vi "4Pi Focus Lock_v2.vi"() -> ()   [LabVIEW 2016]
uses:
  4Pi Focus Lock Controls/4Pi Focus Lock - Notifier Type.ctl
  4Pi Focus Lock Controls/4Pi Focus Lock - Actions.ctl
  <vilib>/vision/Image Controls.llb/IMAQ Image.ctl
  Hardware Configuration/Hardware Configuration Controls/Device Type.ctl
  Hardware Configuration/Hardware Configuration Controls/Device Function.ctl
  Device Library/Cameras/Camera Controls/Generic Camera ROI.ctl
  Device Library/Cameras/Camera Controls/Generic Camera Actions.ctl
  Device Library/Stages/Stages Controls/Stage Actions.ctl
  <vilib>/addons/control/pid/pid.llb/PID (DBL).vi
  <vilib>/addons/control/pid/NI_PID_pid.lvlib
  <vilib>/vision/NI_Vision_Development_Module.lvlib
panel:
  in  "Z Correction Active":bool=TRUE
  in  "Frame Accumulation":u32=1
  in  "Z Drift Threshold (µm)":dbl=2.0
  in  "Z Move Limit (µm)":dbl=2.0
  out "Z Move":bool
  in  "Update Scale Factor":dbl=2.0
  out "dz (µm)":dbl format="%.2f"
  out "dt (s)":dbl format="%.3f"
  out "Measured Z (µm)":dbl=1.0 format="%.3g"
  out "Target Z (µm)":dbl=1.0 format="%.3g"
  out "Stage Position (µm)":dbl=1.0 format="%.2g"
  in  "Quit":bool
  in  "Sample Z Step No.":u32=2
  in  "Sample Z Step Size (µm)":dbl=2.0
  in  "D (Derivative)":dbl
  in  "I (Integral)":dbl
  in  "P (Proportional)":dbl=2.0
  in  "Set Camera ROI":bool
  out "Z Target and Fit Value (µm)":T1(graph)
  in  "Start Lock":bool
  # "PID Control Values"
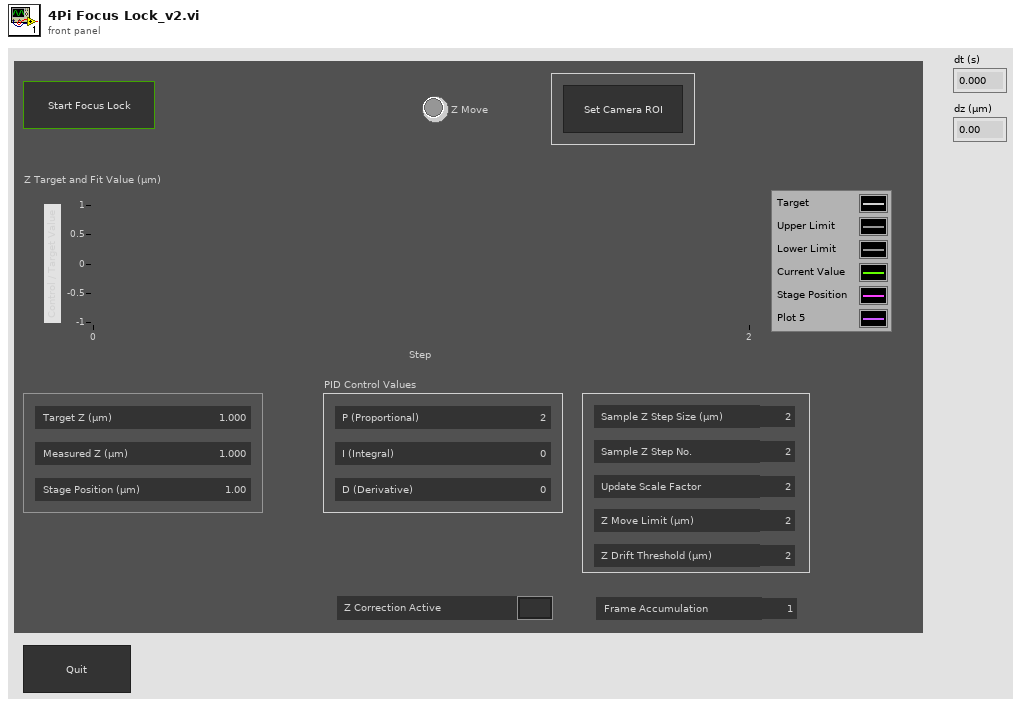
[diagram p1: front panel]
types:
  T1 = cluster{"Target 01":dbl, dbl, dbl, "Current 01":dbl, "Stage Position":dbl}
  T2 = typedef "4Pi Focus Lock - Actions.ctl" = enum16{"Idle", "Start Lock", "Restart Lock", "Get Target Position", "Get Ref Stack", "Cal Ref FFT", "Move To Init Z", "Start Primary Camera", "Get Current Position", "Get Current Position 1", "Get Actual Position", "Check Drift", "Move Z", "Update Plots", "Delay", "Abort", "Exit Loop", "Quit"}
  T3 = typedef "4Pi Focus Lock - Notifier Type.ctl" = cluster{"Actions":T2, "Z Drift Threshold":dbl, "Z Stage Move Limit (µm)":dbl, "Abort If Error":bool, "Z Correction Active":bool, "PID Values":dbl[], "Running?":bool, "Update Delay (ms)":i32, "Z Step Size (µm)":dbl, "Z Step No.":u32, "No. of Frames":u32, "Ref Stack (SGL)":T4[], "Cur Image (SGL)":T4, "CC Image (SGL) ":T4, "Sample Z (µm)":dbl[], "Initial Z Position (µm)":dbl, "Ref FFT Stack (CSG)":T4[], "Tmp Image FFT (CSG) ":T4[]}
  T4 = typedef "IMAQ Image.ctl" = refnum<image>
  T5 = typedef "Image Type" = u32
  T6 = typedef "Device Function.ctl" = enum16{"Primary", "Secondary", "Overview", "Wide Field Drift Correction", "642 nm Excitation", "560 nm Excitation", "940 nm Excitation", "546 nm Excitation", "488 nm Excitation", "405 nm Excitation", "Objective Drift Correction", "4Pi Focus Lock", "4Pi Objective Lock", "Objective XY", "Objective Z", "Sample XY", "Sample Coarse Z", "Sample Z", "4Pi Lower", "4Pi Upper", "Em Small", "Em Large", "Ex Small", "Ex Large", "Mojo", "Adj Cavity", "Line Scanning", "Alert"}
  T7 = typedef "Device Type.ctl" = enum16{"AOTF", "Camera", "Deformable Mirror", "Laser", "Flip Mirror", "Shutter", "Stage", "Waveform", "FPGA", "Email"}
  T8 = typedef "Stage Actions.ctl" = enum16{"Get Position", "MVR", "MOVE", "HALT", "ONTARGET", "ERROR", "REFERENCE", "INIT", "VELOCITY", "STATUS", "EXIT", "HOME", "ZEROPOS", "NANOPOS", "ANALOG", "QUIT"}
  T9 = typedef "Generic Camera Actions.ctl" = enum16{"Status", "Live Preview", "Capture", "Abort", "Set Exposure Time (s)", "Get Exposure Time (s)", "Record Settings", "Set ROI", "Get ROI", "Defect Correction On/Off", "Cooler On/Off", "Fan On/Off", "Quit"}
  T10 = typedef "Generic Camera ROI.ctl" = cluster{"H_Offset":u16, "V_Offset":u16, "H_Width":u16, "V_Width":u16}
  T11 = typedef "Stage Status.ctl" = enum16{"Error", "Abort", "Busy", "On Target"}
  T12 = cluster{"PID Values[0]":dbl, "PID Values[1]":dbl, "PID Values[2]":dbl}
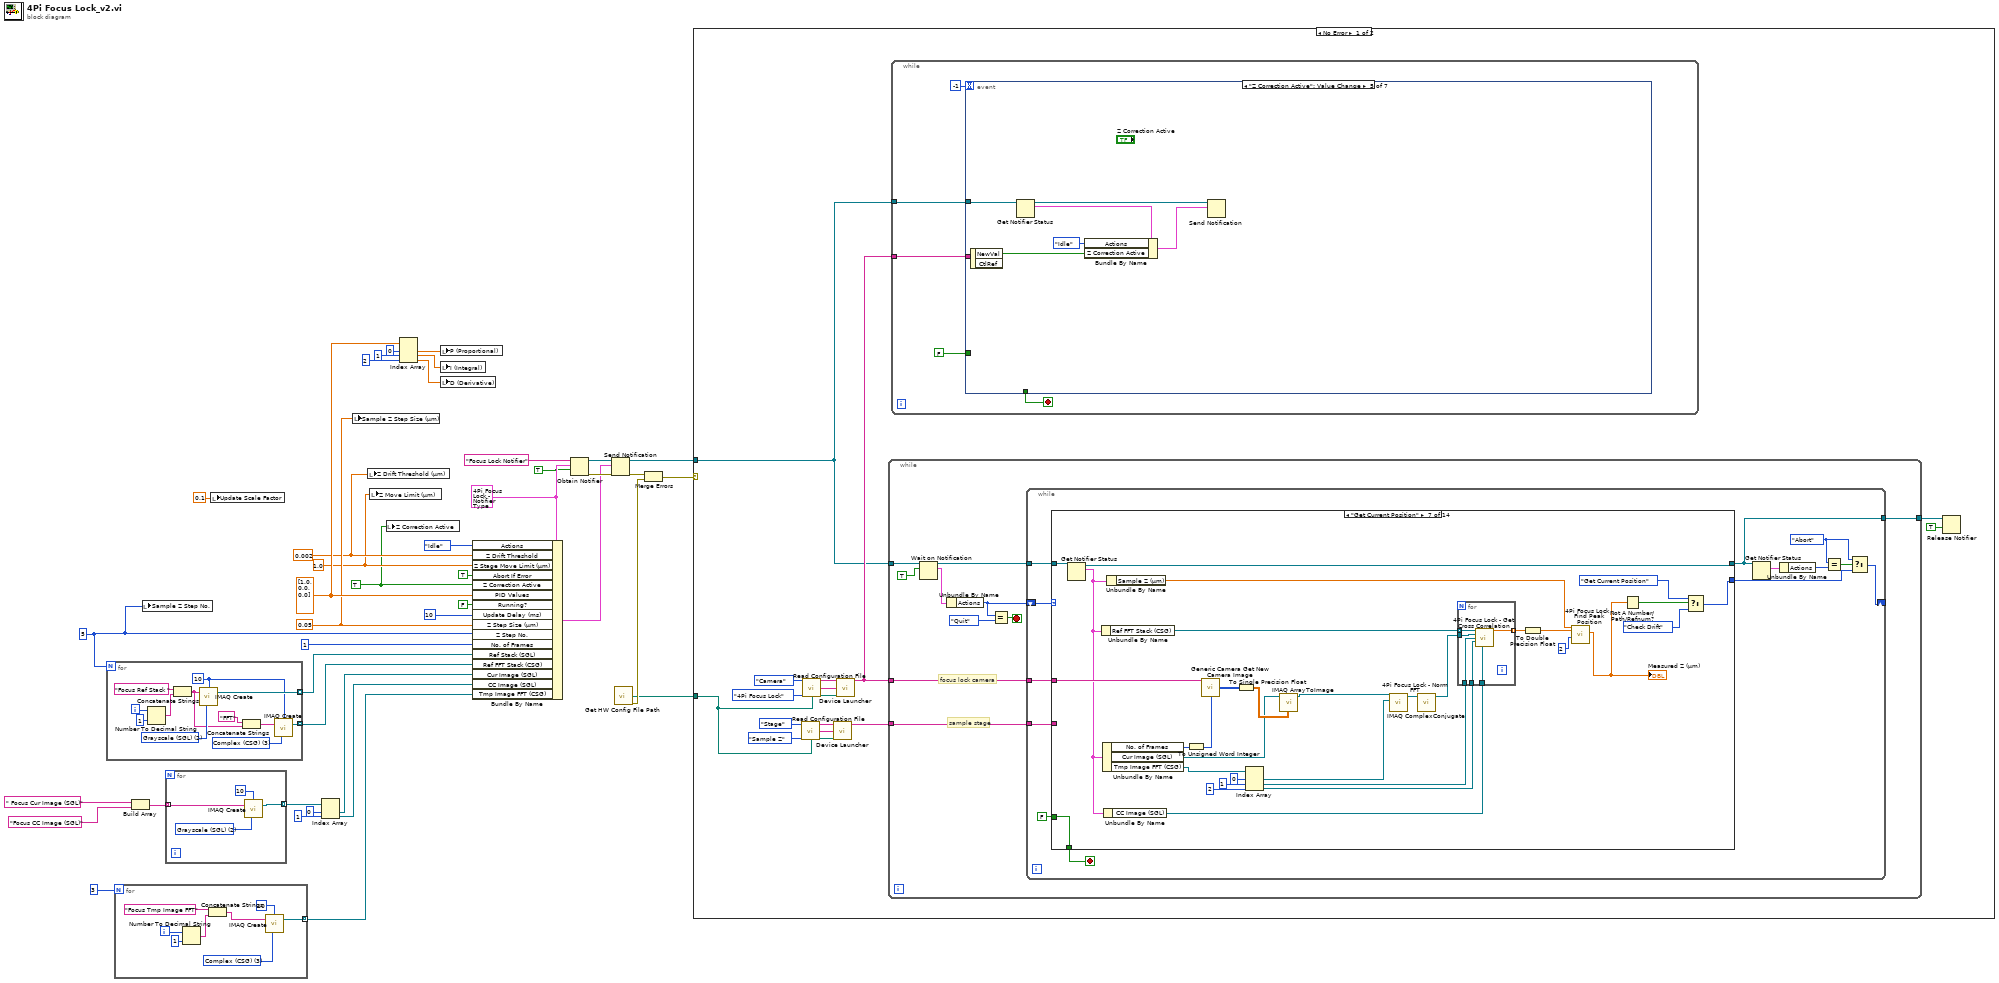
[diagram p0: block diagram]
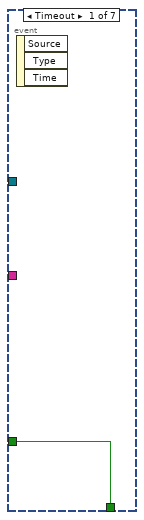
[diagram p2: hidden frame]
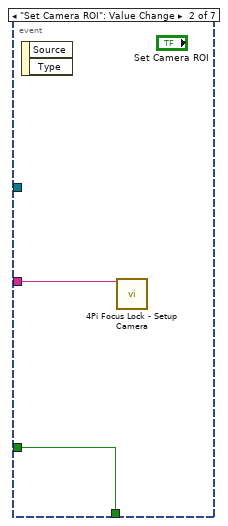
[diagram p3: hidden frame]
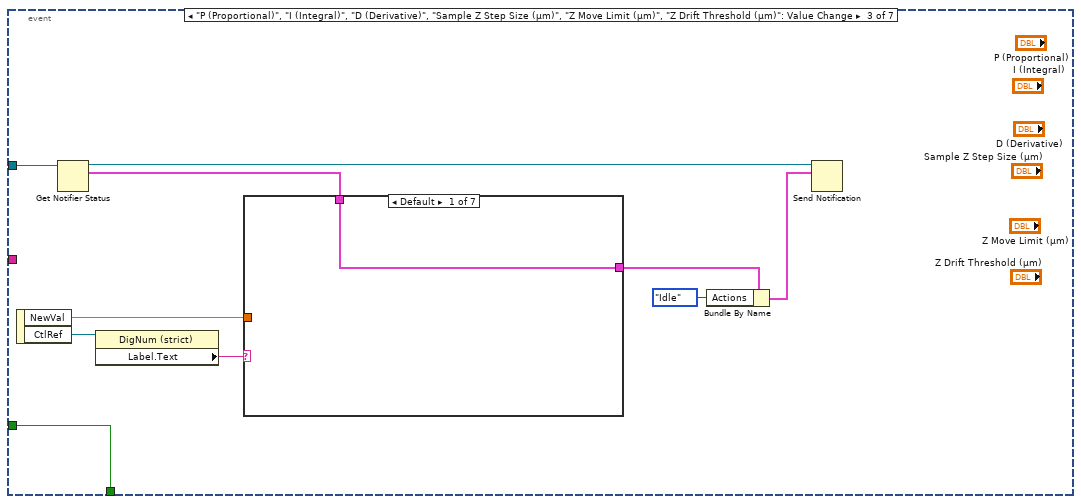
[diagram p4: hidden frame]
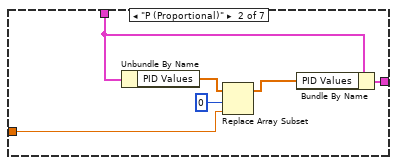
[diagram p5: hidden frame]
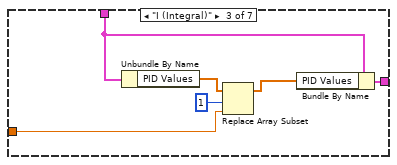
[diagram p6: hidden frame]
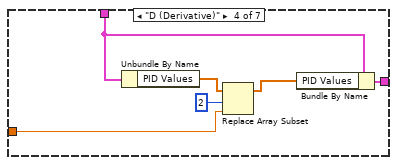
[diagram p7: hidden frame]
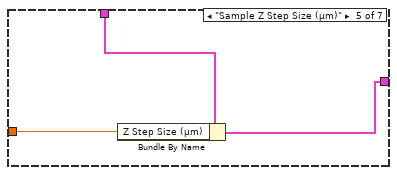
[diagram p8: hidden frame]
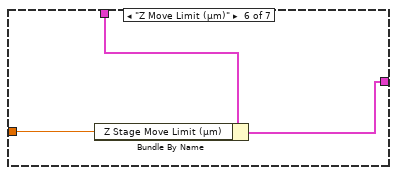
[diagram p9: hidden frame]
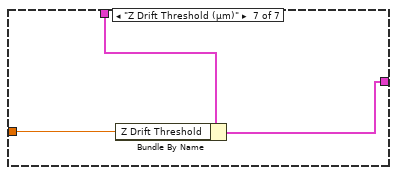
[diagram p10: hidden frame]
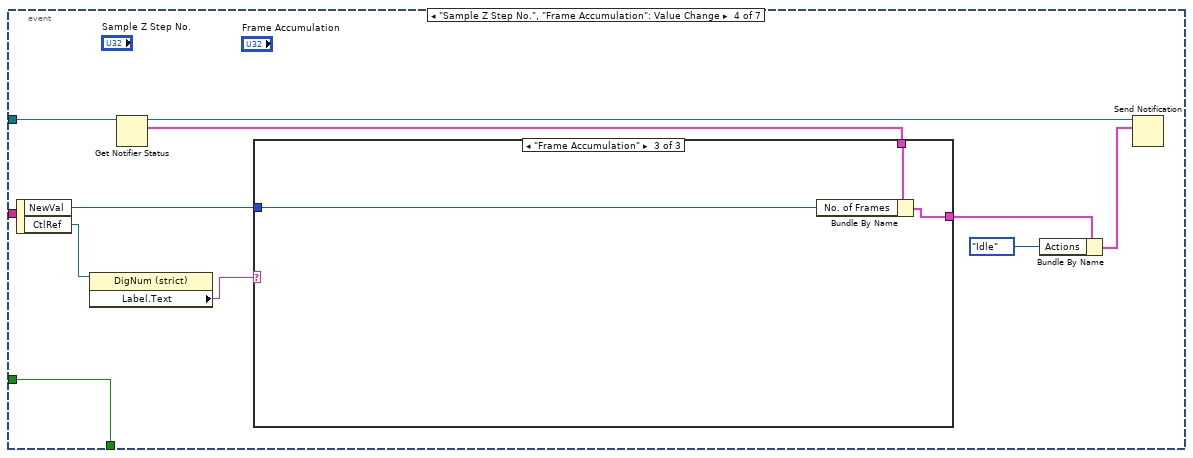
[diagram p11: hidden frame]
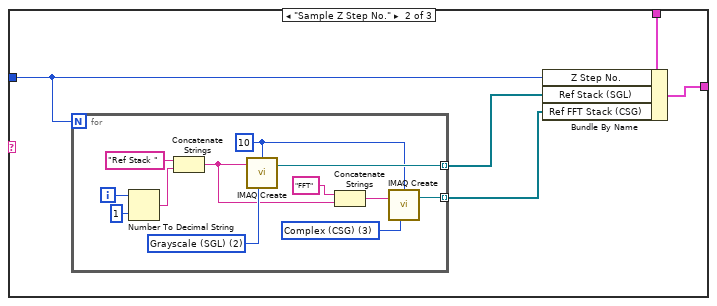
[diagram p13: hidden frame]
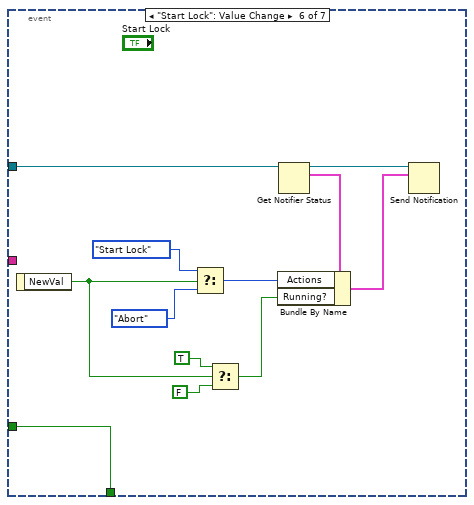
[diagram p14: hidden frame]
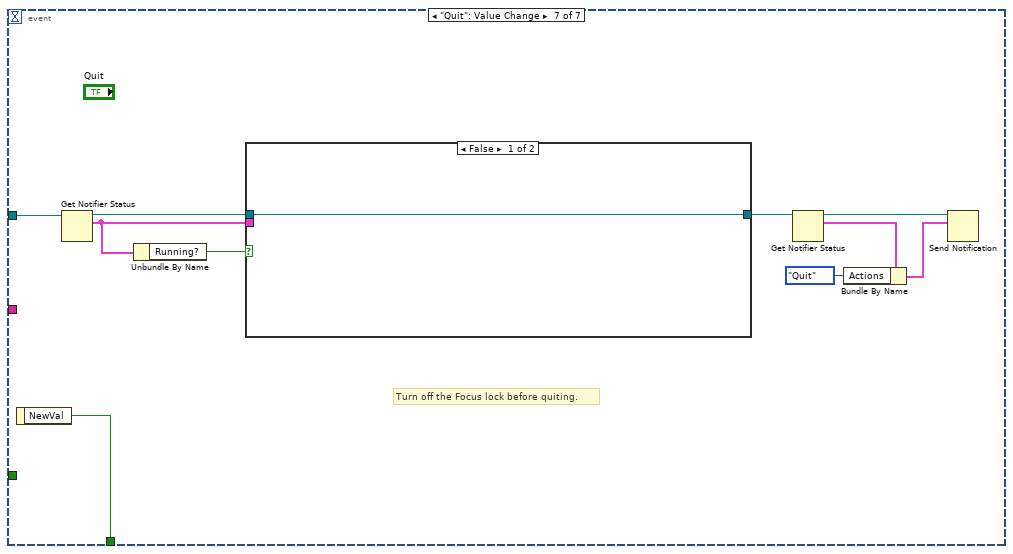
[diagram p15: hidden frame]
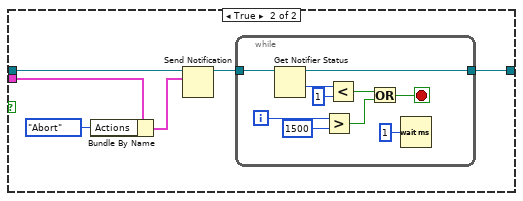
[diagram p16: hidden frame]
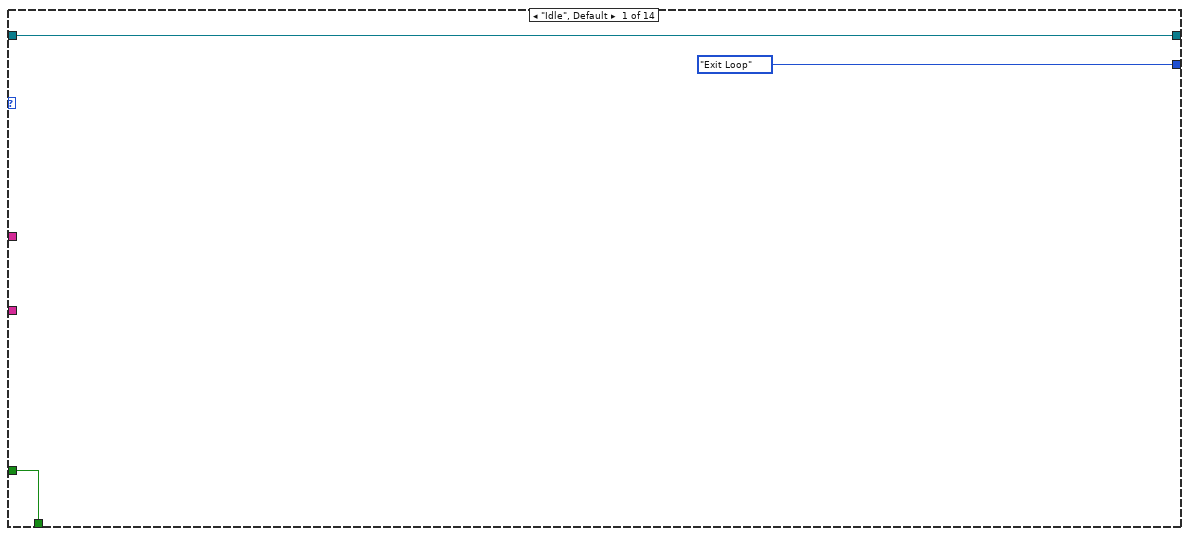
[diagram p17: hidden frame]
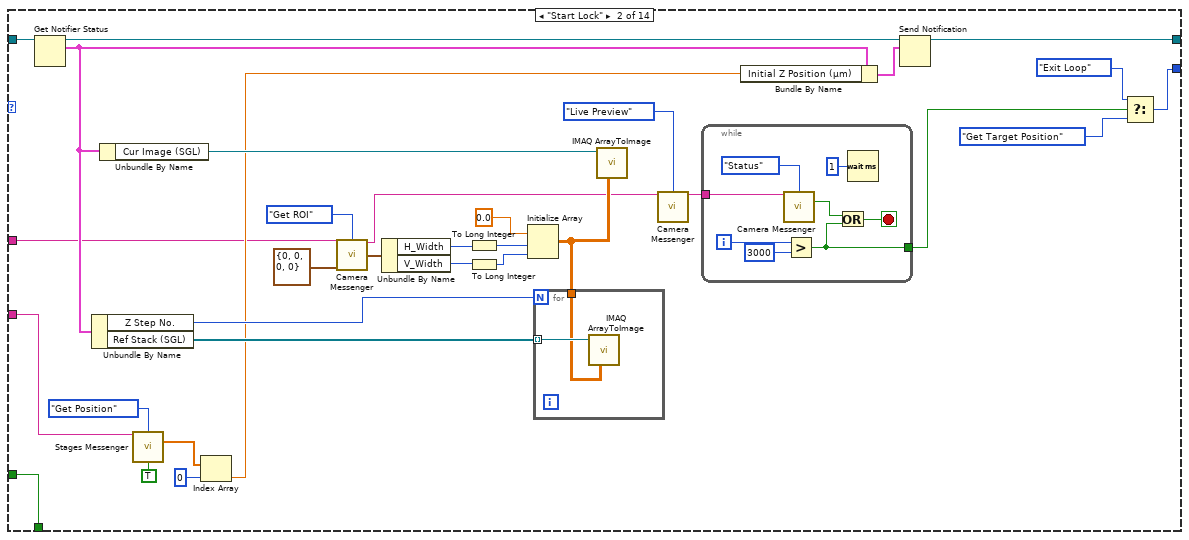
[diagram p18: hidden frame]
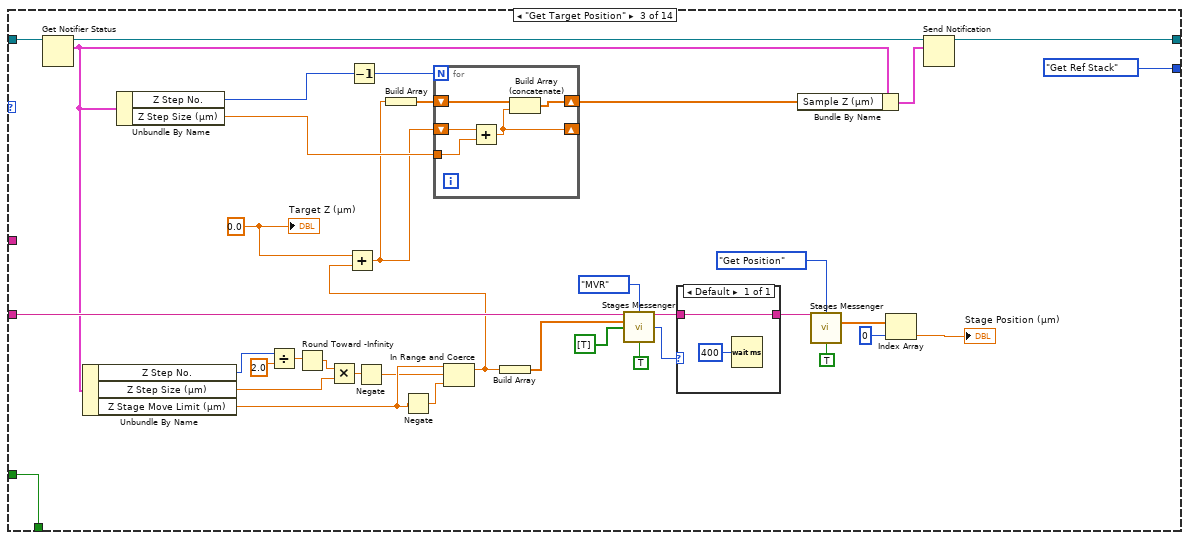
[diagram p19: hidden frame]
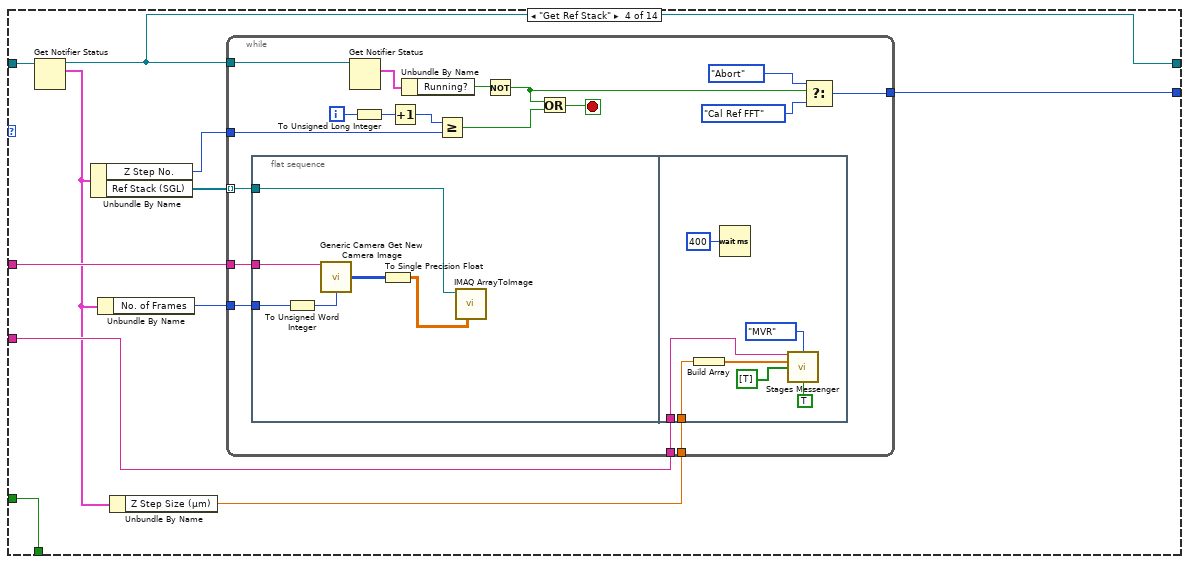
[diagram p20: hidden frame]
diagram:
  w20 = u32 5 ("Z Step No.")
  w27 = 0.05 ("Z Step Size (µm)")
  w31 = dbl[] [1.0, 0.0, 0.0] ("PID Values")
  w1 = TRUE ("Z Correction Active")
  w7 = 1.0 ("Z Stage Move Limit (µm)")
  w8 = 0.002 ("Z Drift Threshold")
  w10 = T3 {"Actions"=enum."Idle", "Z Drift Threshold"=0.05, "Z Stage Move Limit (µm)"=1.0, "Abort If Error"=FALSE, "Z Correction Active"=FALSE, "PID Values"=[], "Running?"=FALSE, "Update Delay (ms)"=0, "Z Step Size (µm)"=2.0, "Z Step No."=2, "No. of Frames"=0, "Ref Stack (SGL)"=[], "Cur Image (SGL)"=refnum, "CC Image (SGL) "=refnum, "Sample Z (µm)"=[], "Initial Z Position (µm)"=0.0, "Ref FFT Stack (CSG)"=[], "Tmp Image FFT (CSG) "=[]} ("4Pi Focus Lock")
  n1 = for {
    N: w20 -> [_]
    tunnel: [w53] -> w19 mode=indexing
    tunnel: [w42] -> w4 mode=indexing
    i -> [w52]
    w47 = T5 3 items=["Grayscale (U8)", "Grayscale (I16)", "Grayscale (SGL)", "Complex (CSG)", "RGB (U32)", "HSL (U32)", "RGB (U64)", "Grayscale (U16)"] ("Image Type")
    w48 = T5 2 items=["Grayscale (U8)", "Grayscale (I16)", "Grayscale (SGL)", "Complex (CSG)", "RGB (U32)", "HSL (U32)", "RGB (U64)", "Grayscale (U16)"] ("Image Type")
    w44 = 10 ("Border Size")
    n2 = Number To Decimal String(number=w52, width (-)=i16 1) -> (decimal integer string=w50:string)
    n3 = Concatenate Strings("Focus Ref Stack " ("string"), w50) -> (w43:string)
    n4 = call "IMAQ Create"("Border Size"=w44, "Image Name"=w43, "Image Type"=w48) -> ("New Image"=w53:T4)  [unwired: 2 in, 1 out]
    n5 = Concatenate Strings("FFT" ("string"), w43) -> (w46:string)
    n6 = call "IMAQ Create"("Border Size"=w44, "Image Name"=w46, "Image Type"=w47) -> ("New Image"=w42:T4)  [unwired: 2 in, 1 out]
  }
  n7 = for {
    N: 3 -> [_]
    tunnel: [w59] -> w2 mode=indexing
    i -> [w55]
    w60 = T5 3 items=["Grayscale (U8)", "Grayscale (I16)", "Grayscale (SGL)", "Complex (CSG)", "RGB (U32)", "HSL (U32)", "RGB (U64)", "Grayscale (U16)"] ("Image Type")
    n8 = Number To Decimal String(number=w55, width (-)=i16 1) -> (decimal integer string=w58:string)
    n9 = Concatenate Strings("Focus Tmp Image FFT" ("Image Name"), w58) -> (w54:string)
    n10 = call "IMAQ Create"("Border Size"=10, "Image Name"=w54, "Image Type"=w60) -> ("New Image"=w59:T4)  [unwired: 2 in, 1 out]
  }
  n11 = Build Array(" Focus Cur Image (SGL)" ("Image Name"), "Focus CC Image (SGL)" ("Image Name")) -> (w14:string[])
  n12 = local write "Sample Z Step No."(w20) -> ()
  n13 = for {
    tunnel: w14 -> [w63] mode=indexing
    tunnel: [w62] -> w13 mode=indexing
    w64 = T5 2 items=["Grayscale (U8)", "Grayscale (I16)", "Grayscale (SGL)", "Complex (CSG)", "RGB (U32)", "HSL (U32)", "RGB (U64)", "Grayscale (U16)"] ("Image Type")
    n14 = call "IMAQ Create"("Border Size"=10, "Image Name"=w63, "Image Type"=w64) -> ("New Image"=w62:T4)  [unwired: 2 in, 1 out]
  }
  n15 = local write "Update Scale Factor"(0.1 ("Update Scale Factor")) -> ()
  n16 = Index Array(array=w13, index #1=0 ("index"), index #2=1 ("index")) -> (element #1=w12:T4, element #2=w11:T4)
  n17 = local write "Sample Z Step Size (µm)"(w27) -> ()
  n18 = local write "Z Drift Threshold (µm)"(w8) -> ()
  n19 = local write "Z Move Limit (µm)"(w7) -> ()
  n20 = local write "Z Correction Active"(w1) -> ()
  n21 = Index Array(array=w31, index #1=0 ("index"), index #2=1 ("index"), index #3=2 ("index")) -> (element #1=w30:dbl, element #2=w29:dbl, element #3=w28:dbl)
  n22 = local write "P (Proportional)"(w30) -> ()
  n23 = local write "I (Integral)"(w29) -> ()
  n24 = local write "D (Derivative)"(w28) -> ()
  n25 = Bundle By Name(cluster=w10, "Actions"=4Pi_Focus_Lock_-_Actions."Idle", "Z Drift Threshold"=w8, "Z Stage Move Limit (µm)"=w7, "Abort If Error"=TRUE, "Z Correction Active"=w1, "PID Values"=w31, "Running?"=FALSE, "Update Delay (ms)"=10, "Z Step Size (µm)"=w27, "Z Step No."=w20, "No. of Frames"=u32 1, "Ref Stack (SGL)"=w19, "Ref FFT Stack (CSG)"=w4, "Cur Image (SGL)"=w12, "CC Image (SGL)"=w11, "Tmp Image FFT (CSG)"=w2) -> (w5:T3)
  n26 = Obtain Notifier(name (unnamed)="Focus Lock Notifier", notification data type=w10, create if not found? (T)=TRUE) -> (notifier out=w36:refnum<notifier>, error out=w35:errorcluster)  [unwired: 1 in, 1 out]
  n27 = Send Notification(notification=w5, notifier=w36, error in (no error)=w35) -> (notifier out=w22:refnum<notifier>, error out=w26:errorcluster)
  n28 = call "Get HW Config File Path.vi"() -> ("File Path"=w24:path, "Error"=w25:errorcluster)  [unwired: 14 in]
  n29 = Merge Errors(w26, w25) -> (w23:errorcluster)
  n30 = case shown="No Error" w23 {
    tunnel: w24 -> [w66 _]
    tunnel: w22 -> [w69 _]
    frame No Error {
      n31 = call "Read Configuration File.vi"("Device Type"=Device_Type."Stage", "Device Function"=Device_Function."Sample Z", "Config File Path"=w66) -> ("Unique Notifier Name"=w76:string, "Device Ports/IDs/Channels"=w74:string[], "Device Engine Path"=w73:path)  [unwired: 9 in, 1 out]
      n32 = call "Read Configuration File.vi"("Device Type"=Device_Type."Camera", "Device Function"=Device_Function."4Pi Focus Lock", "Config File Path"=w66) -> ("Unique Notifier Name"=w81:string, "Device Ports/IDs/Channels"=w80:string[], "Device Engine Path"=w79:path)  [unwired: 9 in, 1 out]
      n33 = call "Device Launcher.vi"("Notifier Name"=w76, "Device Ports/IDs/Channels"=w74, "Device Engine Path"=w73) -> ("Notifier Name"=w71:string)  [unwired: 11 in, 1 out]
      n34 = call "Device Launcher.vi"("Notifier Name"=w81, "Device Ports/IDs/Channels"=w80, "Device Engine Path"=w79) -> ("Notifier Name"=w70:string)  [unwired: 11 in, 1 out]
      n35 = while {
        tunnel: w69 -> [w213]
        tunnel: w70 -> [w207]
        tunnel: w71 -> [w206]
        tunnel: [w204] -> w67
        stop <- w209 stop-if-true
        # "sample stage"
        # "focus lock camera"
        n36 = Wait on Notification(notifier=w213, ignore previous (F)=TRUE) -> (notifier out=w205:refnum<notifier>, notification=w211:T3)  [unwired: 2 in, 2 out]
        n37 = Unbundle By Name(w211) -> ("Actions"=w208:T2)
        n38 = Equal?(x=w208, y=4Pi_Focus_Lock_-_Actions."Quit") -> (x = y?=w209:bool)
        n39 = while {
          tunnel: w207 -> [w225]
          tunnel: w206 -> [w224]
          tunnel: w205 -> [w223]
          shift-right: [w217] -> _
          shift-left: w208 -> [w226]
          tunnel: [w214] -> w204
          stop <- w216 stop-if-true
          w219 = 4Pi_Focus_Lock_-_Actions."Abort" ("y")
          n40 = case shown="\"Get Current Position\"" w226 {
            tunnel: w225 -> [_ w236 _ w325 _ _ w404 w432 _ _ _ w527 _ _]
            tunnel: w224 -> [_ w244 w303 w318 _ w370 _ _ _ w491 w510 _ _ _]
            tunnel: w223 -> [w227 w254 w304 w326 w363 w375 w421 w447 w476 w496 w520 w528 w535 w538]
            tunnel: [4Pi_Focus_Lock_-_Actions."Exit Loop" ("y") w230 4Pi_Focus_Lock_-_Actions."Get Ref Stack" ("y") w319 4Pi_Focus_Lock_-_Actions."Move To Init Z" ("y") 4Pi_Focus_Lock_-_Actions."Get Current Position" ("y") w407 4Pi_Focus_Lock_-_Actions."Check Drift" ("y") w459 w481 4Pi_Focus_Lock_-_Actions."Get Current Position" ("y") 4Pi_Focus_Lock_-_Actions."Exit Loop" ("y") 4Pi_Focus_Lock_-_Actions."Exit Loop" ("y") 4Pi_Focus_Lock_-_Actions."Quit" ("y")] -> w218
            tunnel: [w227 w239 w291 w321 w360 w373 w417 w442 w469 w489 w508 w524 w535 w538] -> w214
            tunnel: [w228 w238 w290 w320 w358 w371 w416 w441 w468 w488 w507 w523 TRUE TRUE] -> w216
            tunnel: FALSE -> [w228 w238 w290 w320 w358 w371 w416 w441 w468 w488 w507 w523 _ _]
            frame "Idle", Default {
            }
            frame "Start Lock" {
              n41 = Get Notifier Status(notifier=w254) -> (notifier out=w240:refnum<notifier>, current notification=w243:T3)  [unwired: 1 in, 3 out]
              n42 = Unbundle By Name(w243) -> ("Z Step No."=w251:u32, "Ref Stack (SGL)"=w250:T4[])
              n43 = Unbundle By Name(w243) -> ("Cur Image (SGL)"=w248:T4)
              n44 = call "Stages Messenger.vi"("Stage Notifier Name"=w244, "Actions"=Stage_Actions."Get Position", "Exit While Busy?"=TRUE) -> ("Positions"=w245:dbl[])  [unwired: 9 in, 3 out]
              n45 = Index Array(array=w245, index=0) -> (element=w242:dbl)
              n46 = call "Camera Messenger.vi"("Notifier Name"=w236, "General Camera Actions"=Generic_Camera_Actions."Get ROI", "Camera ROI"=T10 {"H_Offset"=0, "V_Offset"=0, "H_Width"=0, "V_Width"=0} ("General Camera ROI")) -> ("Notifier Name Dup"=w235:string, "Camera ROI"=w259:T10)  [unwired: 7 in, 4 out]
              n47 = Unbundle By Name(w259) -> ("H_Width"=w258:u16, "V_Width"=w256:u16)
              n48 = To Long Integer(number=w258) -> (32bit integer=w257:i32)
              n49 = To Long Integer(number=w256) -> (32bit integer=w255:i32)
              n50 = Initialize Array(sgl 0.0 ("element"), w257, w255) -> (w249:sgl[][])
              n51 = for {
                N: w251 -> [_]
                tunnel: w249 -> [w270]
                tunnel: w250 -> [w271] mode=indexing
                n52 = call "IMAQ ArrayToImage"("Image Pixels (Float)"=w270, "Image"=w271) -> ()  [unwired: 8 in, 2 out]
              }
              n53 = call "IMAQ ArrayToImage"("Image Pixels (Float)"=w249, "Image"=w248) -> ()  [unwired: 8 in, 2 out]
              n54 = call "Camera Messenger.vi"("Notifier Name"=w235, "General Camera Actions"=Generic_Camera_Actions."Live Preview") -> ("Notifier Name Dup"=w234:string)  [unwired: 8 in, 5 out]
              n55 = while {
                tunnel: w234 -> [w268]
                tunnel: [w263] -> w233
                i -> [w267]
                stop <- w264 stop-if-true
                n56 = call "Camera Messenger.vi"("Notifier Name"=w268, "General Camera Actions"=Generic_Camera_Actions."Status") -> ("Running?"=w265:bool)  [unwired: 8 in, 5 out]
                n57 = Greater?(x=w267, y=3000) -> (0:w263:bool)
                n58 = Or(x=w265, y=w263) -> (x .or. y?=w264:bool)
                n59 = Wait (ms)(milliseconds to wait=u32 1) -> ()  [unwired: 1 out]
              }
              n60 = Bundle By Name(cluster=w243, "Initial Z Position (µm)"=w242) -> (w241:T3)
              n61 = Send Notification(notification=w241, notifier=w240) -> (notifier out=w239:refnum<notifier>)  [unwired: 1 in, 1 out]
              n62 = Select(t=4Pi_Focus_Lock_-_Actions."Exit Loop" ("y"), s=w233, f=4Pi_Focus_Lock_-_Actions."Get Target Position") -> (s? t:f=w230:T2)
            }
            frame "Get Target Position" {
              w297 = 0.0 ("Target Z (µm)")
              n63 = Get Notifier Status(notifier=w304) -> (notifier out=w295:refnum<notifier>, current notification=w300:T3)  [unwired: 1 in, 3 out]
              n64 = Unbundle By Name(w300) -> ("Z Step No."=w289:u32, "Z Step Size (µm)"=w288:dbl, "Z Stage Move Limit (µm)"=w286:dbl)
              n65 = Unbundle By Name(w300) -> ("Z Step No."=w281:u32, "Z Step Size (µm)"=w298:dbl)
              n66 = Divide(x=w289, y=2.0) -> (x/y=w279:dbl)
              n67 = Round Toward -Infinity(1:w279) -> (0:w278:dbl)
              n68 = Multiply(x=w278, y=w288) -> (x*y=w283:dbl)
              n69 = Decrement(x=w281) -> (x-1=w280:u32)
              n70 = Negate(x=w283) -> (-x=w282:dbl)
              n71 = Negate(x=w286) -> (-x=w287:dbl)
              n72 = In Range and Coerce(upper limit=w286, x=w282, lower limit=w287) -> (coerced(x)=w284:dbl)  [unwired: 1 out]
              n73 = Add(x=w297, y=w284) -> (x+y=w285:dbl)
              n74 = Build Array(w285) -> (w299:dbl[])
              n75 = for {
                N: w280 -> [_]
                tunnel: w298 -> [w313]
                shift-right: [w314] -> w296
                shift-left: w299 -> [w315]
                shift-right: [w311] -> _
                shift-left: w285 -> [w312]
                n76 = Add(x=w312, y=w313) -> (x+y=w311:dbl)
                n77 = Build Array (concatenate)(w315, w311) -> (w314:dbl[])
              }
              n78 = Build Array(w284) -> (w301:dbl[])
              n79 = call "Stages Messenger.vi"("Stage Notifier Name"=w303, "Actions"=Stage_Actions."MVR", "Setpoint"=w301, "Axis"=bool[] [TRUE], "Exit While Busy?"=TRUE) -> ("Stage Notifier Name (Dup)"=w276:string, "Status"=w277:T11)  [unwired: 7 in, 2 out]
              n80 = case shown="Default" w277 {
                tunnel: [w309] -> w275
                tunnel: w276 -> [w309]
                frame Default {
                  n81 = Wait (ms)(milliseconds to wait=u32 400) -> ()  [unwired: 1 out]
                }
              }
              n82 = Bundle By Name(cluster=w300, "Sample Z (µm)"=w296) -> (w294:T3)
              n83 = call "Stages Messenger.vi"("Stage Notifier Name"=w275, "Actions"=Stage_Actions."Get Position", "Exit While Busy?"=TRUE) -> ("Positions"=w273:dbl[])  [unwired: 9 in, 3 out]
              n84 = Index Array(array=w273, index=0) -> (element=→"Stage Position (µm)":dbl)
              n85 = Send Notification(notification=w294, notifier=w295) -> (notifier out=w291:refnum<notifier>)  [unwired: 1 in, 1 out]
              "Target Z (µm)" <- w297
            }
            frame "Get Ref Stack" {
              n86 = Get Notifier Status(notifier=w326) -> (notifier out=w321:refnum<notifier>, current notification=w317:T3)  [unwired: 1 in, 3 out]
              n87 = Unbundle By Name(w317) -> ("Z Step No."=w324:u32, "Ref Stack (SGL)"=w323:T4[])
              n88 = Unbundle By Name(w317) -> ("No. of Frames"=w316:u32)
              n89 = Unbundle By Name(w317) -> ("Z Step Size (µm)"=w322:dbl)
              n90 = while {
                tunnel: w325 -> [w344]
                tunnel: w324 -> [w341]
                tunnel: w321 -> [w343]
                tunnel: [w331] -> w319
                tunnel: w323 -> [w330] mode=indexing
                tunnel: w322 -> [w329]
                tunnel: w318 -> [w328]
                tunnel: w316 -> [w327]
                i -> [w340]
                stop <- w336 stop-if-true
                n91 = flat-sequence {
                  tunnel: w344 -> [w348]
                  tunnel: w330 -> [w347]
                  tunnel: w327 -> [w346]
                  tunnel: w329 -> [w352]
                  tunnel: w328 -> [w351]
                  frame #0 {
                    n92 = To Unsigned Word Integer(number=w346) -> (unsigned 16bit integer=w345:u16)
                    n93 = call "Generic Camera Get New Camera Image.vi"("Camera Notifier Name"=w348, "Frames"=w345) -> ("Image - U16"=w350:u16[][])  [unwired: 11 in, 2 out]
                    n94 = To Single Precision Float(number=w350) -> (single precision float=w349:sgl[][])
                    n95 = call "IMAQ ArrayToImage"("Image Pixels (Float)"=w349, "Image"=w347) -> ()  [unwired: 8 in, 2 out]
                  }
                  frame #1 {
                    n96 = Build Array(w352) -> (w356:dbl[])
                    n97 = Wait (ms)(milliseconds to wait=u32 400) -> ()  [unwired: 1 out]
                    n98 = call "Stages Messenger.vi"("Stage Notifier Name"=w351, "Actions"=Stage_Actions."MVR", "Setpoint"=w356, "Axis"=bool[] [TRUE], "Exit While Busy?"=TRUE) -> ()  [unwired: 7 in, 4 out]
                  }
                }
                n99 = Get Notifier Status(notifier=w343) -> (current notification=w335:T3)  [unwired: 1 in, 4 out]
                n100 = To Unsigned Long Integer(number=w340) -> (unsigned 32bit integer=w339:u32)
                n101 = Increment(x=w339) -> (x+1=w342:u32)
                n102 = Unbundle By Name(w335) -> ("Running?"=w338:bool)
                n103 = Greater Or Equal?(x=w342, y=w341) -> (x >= y?=w337:bool)
                n104 = Not(x=w338) -> (.not. x?=w334:bool)
                n105 = Or(x=w334, y=w337) -> (x .or. y?=w336:bool)
                n106 = Select(t=4Pi_Focus_Lock_-_Actions."Abort", s=w334, f=4Pi_Focus_Lock_-_Actions."Cal Ref FFT" ("y")) -> (s? t:f=w331:T2)
              }
            }
            frame "Cal Ref FFT" {
              n107 = Get Notifier Status(notifier=w363) -> (notifier out=w360:refnum<notifier>, current notification=w364:T3)  [unwired: 1 in, 3 out]
              n108 = Unbundle By Name(w364) -> ("Ref Stack (SGL)"=w361:T4[], "Ref FFT Stack (CSG)"=w362:T4[])
              n109 = for {
                tunnel: w362 -> [w365] mode=indexing
                tunnel: w361 -> [w366] mode=indexing
                n110 = call "4Pi Focus Lock - Norm FFT.vi"("FFT Image Dst"=w365, "Image In"=w366) -> ()  [unwired: 8 in, 2 out]
              }
            }
            frame "Move To Init Z" {
              n111 = Get Notifier Status(notifier=w375) -> (notifier out=w373:refnum<notifier>, current notification=w374:T3)  [unwired: 1 in, 3 out]
              n112 = Unbundle By Name(w374) -> ("Initial Z Position (µm)"=w368:dbl)
              n113 = flat-sequence {
                tunnel: w370 -> [w383]
                tunnel: [w382] -> w369
                tunnel: w368 -> [w378]
                tunnel: [w376] -> w367
                tunnel: w369 -> [w387]
                tunnel: w367 -> [w386]
                frame #0 {
                  n114 = call "Stages Messenger.vi"("Stage Notifier Name"=w383, "Actions"=Stage_Actions."Get Position") -> ("Stage Notifier Name (Dup)"=w382:string, "Positions"=w380:dbl[])  [unwired: 10 in, 2 out]
                  n115 = Index Array(array=w380, index=0) -> (element=w379:dbl)
                  n116 = Subtract(x=w378, y=w379) -> (x-y=w377:dbl)
                  n117 = Build Array(w377) -> (w376:dbl[])
                }
                frame #1 {
                  n118 = Wait (ms)(milliseconds to wait=u32 400) -> ()  [unwired: 1 out]
                  n119 = call "Stages Messenger.vi"("Stage Notifier Name"=w387, "Actions"=Stage_Actions."MVR", "Setpoint"=w386, "Axis"=bool[] [TRUE], "Exit While Busy?"=TRUE) -> ()  [unwired: 7 in, 4 out]
                }
              }
            }
            frame "Get Current Position" {
              n120 = Get Notifier Status(notifier=w421) -> (notifier out=w417:refnum<notifier>, current notification=w401:T3)  [unwired: 1 in, 3 out]
              n121 = Unbundle By Name(w401) -> ("Ref FFT Stack (CSG)"=w415:T4[])
              n122 = Unbundle By Name(w401) -> ("No. of Frames"=w392:u32, "Cur Image (SGL)"=w403:T4, "Tmp Image FFT (CSG)"=w397:T4[])
              n123 = Unbundle By Name(w401) -> ("CC Image (SGL)"=w393:T4)
              n124 = Unbundle By Name(w401) -> ("Sample Z (µm)"=w419:dbl[])
              n125 = To Unsigned Word Integer(number=w392) -> (unsigned 16bit integer=w391:u16)
              n126 = call "Generic Camera Get New Camera Image.vi"("Camera Notifier Name"=w404, "Frames"=w391) -> ("Image - U16"=w406:u16[][])  [unwired: 11 in, 2 out]
              n127 = To Single Precision Float(number=w406) -> (single precision float=w405:sgl[][])
              n128 = Index Array(array=w397, index #1=0 ("index"), index #2=1 ("index"), index #3=2 ("index")) -> (element #1=w396:T4, element #2=w395:T4, element #3=w394:T4)
              n129 = call "IMAQ ArrayToImage"("Image Pixels (Float)"=w405, "Image"=w403) -> ("Image Out"=w402:T4)  [unwired: 8 in, 1 out]
              n130 = call "4Pi Focus Lock - Norm FFT.vi"("FFT Image Dst"=w396, "Image In"=w402) -> ("FFT Image Out"=w413:T4)  [unwired: 8 in, 1 out]
              n131 = call "IMAQ ComplexConjugate"("Image Src"=w413) -> ("Image Dst Out"=w412:T4)  [unwired: 3 in, 1 out]
              n132 = for {
                tunnel: w393 -> [w427]
                tunnel: [w426] -> w420 mode=indexing
                tunnel: w412 -> [w425]
                tunnel: w415 -> [w424] mode=indexing
                tunnel: w394 -> [w423]
                tunnel: w395 -> [w422]
                n133 = call "4Pi Focus Lock - Get Cross Correlation.vi"("Ref FFT image"=w424, "Cur FFT Image"=w425, "FFT CC image"=w422, "iFFT image"=w423, "CC image"=w427) -> ("Max CC"=w426:sgl)  [unwired: 9 in, 1 out]
              }
              n134 = To Double Precision Float(number=w420) -> (double precision float=w414:dbl[])
              n135 = call "4Pi Focus Lock - Find Peak Position.vi"("Fit Size"=2, "y"=w414, "x"=w419) -> ("Coerced Peak Position"=w411:dbl)  [unwired: 7 in, 1 out]
              "Measured Z (µm)" <- w411
              n136 = Not A Number/Path/Refnum?(number/path/refnum=w411) -> (NaN/Path/Refnum?=w410:bool)
              n137 = Select(t=4Pi_Focus_Lock_-_Actions."Get Current Position", s=w410, f=4Pi_Focus_Lock_-_Actions."Check Drift" ("y")) -> (s? t:f=w407:T2)
            }
            frame "Get Current Position 1" {
              n138 = Get Notifier Status(notifier=w447) -> (notifier out=w442:refnum<notifier>, current notification=w446:T3)  [unwired: 1 in, 3 out]
              n139 = Unbundle By Name(w446) -> ("No. of Frames"=w429:u32, "Cur Image (SGL)"=w431:T4, "CC Image (SGL)"=w437:T4)
              n140 = Unbundle By Name(w446) -> ("Sample Z (µm)"=w445:dbl[])
              n141 = Unbundle By Name(w446) -> ("Ref Stack (SGL)"=w440:T4[])
              n142 = To Unsigned Word Integer(number=w429) -> (unsigned 16bit integer=w428:u16)
              n143 = call "Generic Camera Get New Camera Image.vi"("Camera Notifier Name"=w432, "Frames"=w428) -> ("Image - U16"=w434:u16[][])  [unwired: 11 in, 2 out]
              n144 = To Single Precision Float(number=w434) -> (single precision float=w433:sgl[][])
              n145 = call "IMAQ ArrayToImage"("Image Pixels (Float)"=w433, "Image"=w431) -> ("Image Out"=w430:T4)  [unwired: 8 in, 1 out]
              n146 = call "4Pi Focus Lock - Img Norm.vi"("Image In"=w430) -> ("Image Dst Out"=w438:T4)  [unwired: 9 in, 1 out]
              n147 = for {
                tunnel: w440 -> [w458] mode=indexing
                tunnel: w438 -> [w456]
                tunnel: w437 -> [w455]
                tunnel: [w454] -> w436 mode=indexing
                n148 = call "4Pi Focus Lock - Img Norm.vi"("Image In"=w458) -> ("Image Dst Out"=w457:T4)  [unwired: 9 in, 1 out]
                n149 = call "IMAQ Multiply"("Image Src A"=w457, "Image Dst"=w455, "Image Src B"=w456) -> ("Image Dst Out"=w453:T4)  [unwired: 4 in, 1 out]
                n150 = call "IMAQ ImageToArray"("Image"=w453) -> ("Image Pixels (Float)"=w452:sgl[][])  [unwired: 3 in, 4 out]
                n151 = Add Array Elements(numeric array=w452) -> (sum=w450:sgl)
                n152 = Array Size(array=w452) -> (size(s)=w451:i32[])
                n153 = Multiply Array Elements(1:w451) -> (0:w449:i32)
                n154 = To Double Precision Float(number=w449) -> (double precision float=w448:dbl)
                n155 = Divide(x=w450, y=w448) -> (x/y=w454:dbl)
              }
              n156 = To Double Precision Float(number=w436) -> (double precision float=w439:dbl[])
              n157 = call "4Pi Focus Lock - Find Peak Position.vi"("Fit Size"=2, "y"=w439, "x"=w445) -> ("Coerced Peak Position"=w435:dbl)  [unwired: 7 in, 1 out]
              n158 = local write "Measured Z (µm)"(w435) -> ()
            }
            frame "Check Drift" {
              n159 = Get Notifier Status(notifier=w476) -> (notifier out=w469:refnum<notifier>, current notification=w475:T3)  [unwired: 1 in, 3 out]
              n160 = Unbundle By Name(w475) -> ("Z Correction Active"=w462:bool, "Z Drift Threshold"=w470:dbl, "PID Values"=w474:dbl[])
              n161 = local read "Measured Z (µm)"() -> (w465:dbl)
              n162 = local read "Target Z (µm)"() -> (w466:dbl)
              n163 = Array To Cluster(array=w474) -> (cluster=w473:T12)
              n164 = Subtract(x=w466, y=w465) -> (x-y=w467:dbl)
              n165 = call-poly <vilib>:"PID.vi"("PID gains"=w473, "process variable"=w465, "setpoint"=w466) -> ("dt out (s)"=→"dt (s)":dbl, "output"=→"dz (µm)":dbl)  [unwired: 7 in]
              n166 = Absolute Value(x=w467) -> (abs(x)=w464:dbl)
              n167 = Greater?(x=w464, y=w470) -> (0:w463:bool)
              n168 = And(x=w462, y=w463) -> (x .and. y?=w461:bool)
              n169 = case shown="True" w461 {
                tunnel: [4Pi_Focus_Lock_-_Actions."Update Plots" ("y") 4Pi_Focus_Lock_-_Actions."Move Z" ("y")] -> w459
                tunnel: [FALSE TRUE] -> w460
                frame False {
                }
                frame True {
                }
              }
              "Z Move" <- w460
            }
            frame "Move Z" {
              n170 = Get Notifier Status(notifier=w496) -> (notifier out=w489:refnum<notifier>, current notification=w495:T3)  [unwired: 1 in, 3 out]
              n171 = Unbundle By Name(w495) -> ("Z Stage Move Limit (µm)"=w493:dbl)
              n172 = local read "dz (µm)"() -> (w494:dbl)
              n173 = Multiply(x=w494, y="Update Scale Factor") -> (x*y=w487:dbl)
              n174 = Absolute Value(x=w487) -> (abs(x)=w492:dbl)
              n175 = Greater?(x=w493, y=w492) -> (0:w483:bool)
              n176 = local read "Z Move"() -> (w485:bool)
              n177 = And(x=w483, y=w485) -> (x .and. y?=w486:bool)
              n178 = case shown="True" w486 {
                tunnel: w487 -> [_ w500]
                tunnel: w491 -> [_ w499]
                frame False {
                }
                frame True {
                  n179 = Build Array(w500) -> (w504:dbl[])
                  n180 = call "Stages Messenger.vi"("Stage Notifier Name"=w499, "Actions"=Stage_Actions."MVR", "Setpoint"=w504, "Axis"=bool[] [TRUE], "Exit While Busy?"=TRUE) -> ("Positions"=w502:dbl[])  [unwired: 7 in, 3 out]
                  n181 = Wait (ms)(milliseconds to wait=u32 50) -> ()  [unwired: 1 out]
                  n182 = Index Array(array=w502, index=0) -> ()  [unwired: 1 out]
                }
              }
              n183 = Select(t=4Pi_Focus_Lock_-_Actions."Update Plots" ("y"), s=w483, f=4Pi_Focus_Lock_-_Actions."Abort") -> (s? t:f=w481:T2)
            }
            frame "Update Plots" {
              n184 = Get Notifier Status(notifier=w520) -> (notifier out=w508:refnum<notifier>, current notification=w518:T3)  [unwired: 1 in, 3 out]
              n185 = Unbundle By Name(w518) -> ("Z Drift Threshold"=w519:dbl)
              n186 = Unbundle By Name(w518) -> ("Initial Z Position (µm)"=w517:dbl)
              n187 = call "Stages Messenger.vi"("Stage Notifier Name"=w510, "Actions"=Stage_Actions."Get Position", "Exit While Busy?"=TRUE) -> ("Positions"=w511:dbl[])  [unwired: 9 in, 3 out]
              n188 = local read "Measured Z (µm)"() -> (w521:dbl)
              n189 = local read "Target Z (µm)"() -> (w522:dbl)
              n190 = Index Array(array=w511, index=0) -> (element=w509:dbl)
              n191 = local write "Stage Position (µm)"(w509) -> ()
              n192 = Subtract(x=w509, y=w517) -> (x-y=w516:dbl)
              n193 = call "4Pi Focus Lock - Values Organize Plot Data.vi"("Target 01"=w522, "Value Limit"=w519, "Current 01"=w521, "Stage Position"=w516) -> ("output cluster"=→"Z Target and Fit Value (µm)":T1)  [unwired: 11 in]
            }
            frame "Abort" {
              n194 = Get Notifier Status(notifier=w528) -> (notifier out=w533:refnum<notifier>, current notification=w532:T3)  [unwired: 1 in, 3 out]
              n195 = call "Camera Messenger.vi"("Notifier Name"=w527, "General Camera Actions"=Generic_Camera_Actions."Abort") -> ()  [unwired: 8 in, 6 out]
              n196 = Bundle By Name(cluster=w532, "Running?"=FALSE, "Actions"=4Pi_Focus_Lock_-_Actions."Exit Loop") -> (w530:T3)
              n197 = Send Notification(notification=w530, notifier=w533) -> (notifier out=w524:refnum<notifier>)  [unwired: 1 in, 1 out]
            }
            frame "Exit Loop" {
            }
            frame "Quit" {
              n198 = Get Notifier Status(notifier=w538) -> (current notification=w544:T3)  [unwired: 1 in, 4 out]
              n199 = Unbundle By Name(w544) -> ("Ref Stack (SGL)"=w543:T4[], "Cur Image (SGL)"=w542:T4, "Tmp Image FFT (CSG)"=w541:T4[], "CC Image (SGL)"=w540:T4, "Ref FFT Stack (CSG)"=w537:T4[])
              n200 = Build Array (concatenate)(w543, w542, w541, w540, w537) -> (w539:T4[])
              n201 = for {
                tunnel: w539 -> [w547] mode=indexing
                n202 = call "IMAQ Dispose"("Image"=w547) -> ()  [unwired: 5 in, 1 out]
              }
            }
          }
          n203 = Get Notifier Status(notifier=w214) -> (current notification=w222:T3)  [unwired: 1 in, 4 out]
          n204 = Unbundle By Name(w222) -> ("Actions"=w221:T2)
          n205 = Equal?(x=w219, y=w221) -> (x = y?=w220:bool)
          n206 = Select(t=w219, s=w220, f=w218) -> (s? t:f=w217:T2)
        }
      }
      n207 = while {
        tunnel: w70 -> [w86]
        tunnel: w69 -> [w85]
        stop <- w84 stop-if-true
        n208 = event shown="[4] \"Z Correction Active\": Value Change" {
          selector: _ -> [_ _ _ _ _ _ _]
          dyn-events: _ -> [_ _ _ _ _ _ _]
          timeout: -1 -> [_ _ _ _ _ _ _]
          tunnel: w86 -> [_ w89 _ _ _ _ _]
          tunnel: w85 -> [_ _ w99 w137 w164 w175 w179]
          tunnel: [w87 w88 w90 w134 _ w169 w177] -> w84
          tunnel: FALSE ("NewVal") -> [w87 w88 w90 w134 _ w169 _]
          event Timeout {
            n209 = event-data() -> ()  [unwired: 1 in, 3 out]
          }
          event "Set Camera ROI": Value Change {
            n210 = event-data() -> ()  [unwired: 1 in, 2 out]
            n211 = call "4Pi Focus Lock - Setup Camera.vi"("Camera Notifier Name"=w89) -> ()  [unwired: 14 in, 1 out]
          }
          event "P (Proportional)", "I (Integral)", "D (Derivative)", "Sample Z Step Size (µm)", "Z Move Limit (µm)", "Z Drift Threshold (µm)": Value Change {
            n212 = event-data() -> ("NewVal"=w94:dbl, "CtlRef"=w96:refnum<vi>)  [unwired: 1 in]
            n213 = Get Notifier Status(notifier=w99) -> (notifier out=w98:refnum<notifier>, current notification=w97:T3)  [unwired: 1 in, 3 out]
            n214 = property class="DigNum (strict)"(reference=w96) -> ("Label.Text"=w95:string)  [unwired: 1 in, 2 out]
            n215 = case shown="Default" w95 {
              tunnel: w97 -> [w100 w103 w109 w115 w121 w124 w127]
              tunnel: w94 -> [_ w104 w110 w116 w120 w123 w126]
              tunnel: [w100 w101 w107 w113 w119 w122 w125] -> w93
              frame Default {
              }
              frame "P (Proportional)" {
                n216 = Unbundle By Name(w103) -> ("PID Values"=w105:dbl[])
                n217 = Replace Array Subset(array=w105, new element=w104, index=0) -> (w102:dbl[])
                n218 = Bundle By Name(cluster=w103, "PID Values"=w102) -> (w101:T3)
              }
              frame "I (Integral)" {
                n219 = Unbundle By Name(w109) -> ("PID Values"=w111:dbl[])
                n220 = Replace Array Subset(array=w111, new element=w110, index=1) -> (w108:dbl[])
                n221 = Bundle By Name(cluster=w109, "PID Values"=w108) -> (w107:T3)
              }
              frame "D (Derivative)" {
                n222 = Unbundle By Name(w115) -> ("PID Values"=w117:dbl[])
                n223 = Replace Array Subset(array=w117, new element=w116, index=2) -> (w114:dbl[])
                n224 = Bundle By Name(cluster=w115, "PID Values"=w114) -> (w113:T3)
              }
              frame "Sample Z Step Size (µm)" {
                n225 = Bundle By Name(cluster=w121, "Z Step Size (µm)"=w120) -> (w119:T3)
              }
              frame "Z Move Limit (µm)" {
                n226 = Bundle By Name(cluster=w124, "Z Stage Move Limit (µm)"=w123) -> (w122:T3)
              }
              frame "Z Drift Threshold (µm)" {
                n227 = Bundle By Name(cluster=w127, "Z Drift Threshold"=w126) -> (w125:T3)
              }
            }
            n228 = Bundle By Name(cluster=w93, "Actions"=4Pi_Focus_Lock_-_Actions."Idle") -> (w91:T3)
            n229 = Send Notification(notification=w91, notifier=w98) -> ()  [unwired: 1 in, 2 out]
          }
          event "Sample Z Step No.", "Frame Accumulation": Value Change {
            n230 = event-data() -> ("NewVal"=w133:u32, "CtlRef"=w129:refnum<vi>)  [unwired: 1 in]
            n231 = property class="DigNum (strict)"(reference=w129) -> ("Label.Text"=w128:string)  [unwired: 1 in, 2 out]
            n232 = Get Notifier Status(notifier=w137) -> (notifier out=w135:refnum<notifier>, current notification=w136:T3)  [unwired: 1 in, 3 out]
            n233 = case shown="\"Frame Accumulation\"" w128 {
              tunnel: w136 -> [w138 w143 w158]
              tunnel: [w138 w142 w156] -> w132
              tunnel: w133 -> [_ w141 w157]
              frame Default {
              }
              frame "Sample Z Step No." {
                n234 = for {
                  N: w141 -> [_]
                  tunnel: [w155] -> w140 mode=indexing
                  tunnel: [w144] -> w139 mode=indexing
                  i -> [w154]
                  w145 = T5 3 items=["Grayscale (U8)", "Grayscale (I16)", "Grayscale (SGL)", "Complex (CSG)", "RGB (U32)", "HSL (U32)", "RGB (U64)", "Grayscale (U16)"] ("Image Type")
                  w150 = T5 2 items=["Grayscale (U8)", "Grayscale (I16)", "Grayscale (SGL)", "Complex (CSG)", "RGB (U32)", "HSL (U32)", "RGB (U64)", "Grayscale (U16)"] ("Image Type")
                  w146 = 10 ("Border Size")
                  n235 = Number To Decimal String(number=w154, width (-)=i16 1) -> (decimal integer string=w152:string)
                  n236 = Concatenate Strings("Ref Stack " ("string"), w152) -> (w148:string)
                  n237 = call "IMAQ Create"("Border Size"=w146, "Image Name"=w148, "Image Type"=w150) -> ("New Image"=w155:T4)  [unwired: 2 in, 1 out]
                  n238 = Concatenate Strings("FFT" ("string"), w148) -> (w147:string)
                  n239 = call "IMAQ Create"("Border Size"=w146, "Image Name"=w147, "Image Type"=w145) -> ("New Image"=w144:T4)  [unwired: 2 in, 1 out]
                }
                n240 = Bundle By Name(cluster=w143, "Z Step No."=w141, "Ref Stack (SGL)"=w140, "Ref FFT Stack (CSG)"=w139) -> (w142:T3)
              }
              frame "Frame Accumulation" {
                n241 = Bundle By Name(cluster=w158, "No. of Frames"=w157) -> (w156:T3)
              }
            }
            n242 = Bundle By Name(cluster=w132, "Actions"=4Pi_Focus_Lock_-_Actions."Idle") -> (w130:T3)
            n243 = Send Notification(notification=w130, notifier=w135) -> ()  [unwired: 1 in, 2 out]
          }
          event "Z Correction Active": Value Change {
            n244 = event-data() -> ("NewVal"=w162:bool)  [unwired: 1 in, 1 out]
            n245 = Get Notifier Status(notifier=w164) -> (notifier out=w160:refnum<notifier>, current notification=w163:T3)  [unwired: 1 in, 3 out]
            n246 = Bundle By Name(cluster=w163, "Actions"=4Pi_Focus_Lock_-_Actions."Idle", "Z Correction Active"=w162) -> (w159:T3)
            n247 = Send Notification(notification=w159, notifier=w160) -> ()  [unwired: 1 in, 2 out]
          }
          event "Start Lock": Value Change {
            n248 = event-data() -> ("NewVal"=w167:bool)  [unwired: 1 in]
            n249 = Select(t=4Pi_Focus_Lock_-_Actions."Start Lock", s=w167, f=4Pi_Focus_Lock_-_Actions."Abort" ("t")) -> (s? t:f=w172:T2)
            n250 = Select(t=TRUE ("Running?"), s=w167, f=FALSE) -> (s? t:f=w165:bool)
            n251 = Get Notifier Status(notifier=w175) -> (notifier out=w176:refnum<notifier>, current notification=w174:T3)  [unwired: 1 in, 3 out]
            n252 = Bundle By Name(cluster=w174, "Actions"=w172, "Running?"=w165) -> (w173:T3)
            n253 = Send Notification(notification=w173, notifier=w176) -> ()  [unwired: 1 in, 2 out]
          }
          event "Quit": Value Change {
            # "Turn off the Focus lock before quiting."
            n254 = event-data() -> ("NewVal"=w177:bool)  [unwired: 1 in]
            n255 = Get Notifier Status(notifier=w179) -> (notifier out=w182:refnum<notifier>, current notification=w180:T3)  [unwired: 1 in, 3 out]
            n256 = Unbundle By Name(w180) -> ("Running?"=w183:bool)
            n257 = case shown="False" w183 {
              tunnel: w182 -> [w187 w192]
              tunnel: [w187 w189] -> w181
              tunnel: w180 -> [_ w193]
              frame False {
              }
              frame True {
                n258 = Bundle By Name(cluster=w193, "Actions"=4Pi_Focus_Lock_-_Actions."Abort") -> (w191:T3)
                n259 = Send Notification(notification=w191, notifier=w192) -> (notifier out=w190:refnum<notifier>)  [unwired: 1 in, 1 out]
                n260 = while {
                  tunnel: w190 -> [w203]
                  tunnel: [w198] -> w189
                  i -> [w197]
                  stop <- w199 stop-if-true
                  n261 = Get Notifier Status(notifier=w203) -> (notifier out=w198:refnum<notifier>, # waiting=w202:i32)  [unwired: 1 in, 3 out]
                  n262 = Greater?(x=w197, y=1500) -> (0:w195:bool)
                  n263 = Less?(x=w202, y=1) -> (x < y?=w200:bool)
                  n264 = Or(x=w200, y=w195) -> (x .or. y?=w199:bool)
                  n265 = Wait (ms)(milliseconds to wait=u32 1) -> ()  [unwired: 1 out]
                }
              }
            }
            n266 = Get Notifier Status(notifier=w181) -> (notifier out=w185:refnum<notifier>, current notification=w186:T3)  [unwired: 1 in, 3 out]
            n267 = Bundle By Name(cluster=w186, "Actions"=4Pi_Focus_Lock_-_Actions."Quit") -> (w184:T3)
            n268 = Send Notification(notification=w184, notifier=w185) -> ()  [unwired: 1 in, 2 out]
          }
        }
      }
      n269 = Release Notifier(notifier=w67, force destroy? (F)=TRUE) -> ()  [unwired: 1 in, 3 out]
    }
    frame Error {
    }
  }
